vi "Command Formation And Communication.vi"(8 "error in (no error)":errorcluster, 9 "Command":string, 10 "Platform Slot Number":i16 min=-1 max=255, 11 "VISA resource name":refnum<visa-resource-name>) -> (0 "error out":errorcluster, 2 "Response":string, 3 "VISA resource name out":refnum<visa-resource-name>)   [LabVIEW 2018, in "LTB-1.lvlib" / "3150.lvlib"]
doc: "Responsible for communication with the device, sending the command and receiving the output, adding LINS keyword if command belongs to module-specific. Calls the error query based on the mode of communication and logged into the error cluster using Merge Error.vi if any error encounters."
uses:
  3150.lvlib
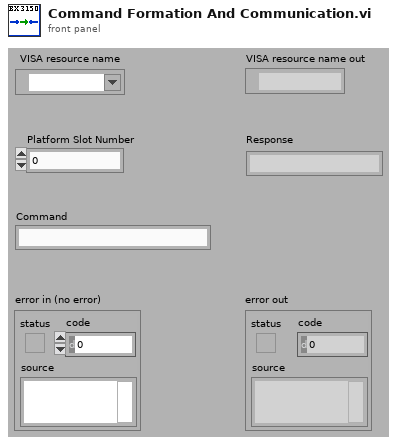
[diagram p1: front panel]
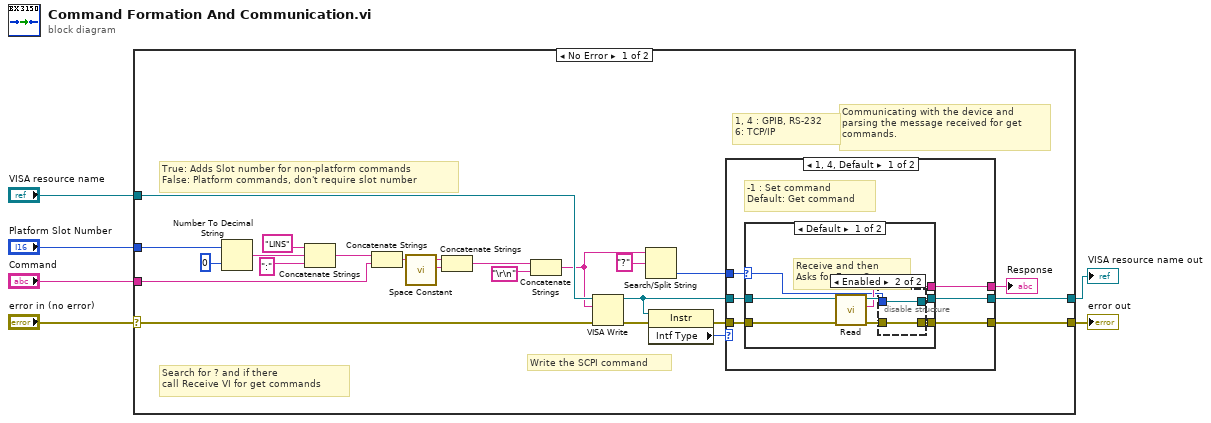
[diagram p0: block diagram]
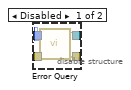
[diagram p2: hidden frame]
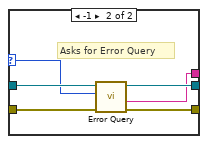
[diagram p3: hidden frame]
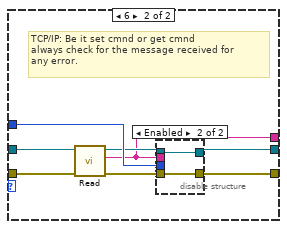
[diagram p4: hidden frame]
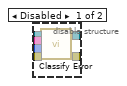
[diagram p5: hidden frame]
diagram:
  n1 = case shown="No Error" "error in (no error)" {
    selector: "error in (no error)" -> [w27 w73]
    tunnel: "VISA resource name" -> [w29 w74]
    tunnel: [w16 w74] -> w4
    tunnel: "Command" -> [w28 _]
    tunnel: [w15 w73] -> w1
    tunnel: "Platform Slot Number" -> [w26 _]
    frame No Error {
      # "1, 4 : GPIB, RS-232\n6: TCP/IP"
      # "Write the SCPI command"
      # "Search for ? and if there\ncall Receive VI for get commands"
      # "Communicating with the device and \nparsing the message received for get\ncommands."
      # "True: Adds Slot number for non-platform commands\nFalse: Platform commands, don't require slot number"
      n2 = Number To Decimal String(number=w26, width (-)=0) -> (decimal integer string=w9:string)
      n3 = Concatenate Strings("LINS", w9, ":" ("string")) -> (w10:string)
      n4 = Concatenate Strings(w10, w28) -> (w11:string)
      n5 = call <vilib>:"Space Constant.vi"() -> ("String"=w7:string)
      n6 = Concatenate Strings(w11, w7) -> (w25:string)
      n7 = Concatenate Strings(w25, "\r\n") -> (w22:string)
      n8 = VISA Write(VISA resource name=w29, write buffer=w22, error in (no error)=w27) -> (VISA resource name out=w19:refnum<visa-resource-name>, error out=w17:errorcluster)  [unwired: 1 out]
      n9 = Search/Split String(string=w22, search string/char (-)="?") -> (offset of match=w21:i32)  [unwired: 3 out]
      n10 = property class="Instr"(reference=w19, error in=w17) -> (error out=w18:errorcluster, "Intf Type"=w20:u16)  [unwired: 1 out]
      n11 = case shown="1, 4, Default" w20 {
        tunnel: w21 -> [w35 w62]
        tunnel: w19 -> [w33 w64]
        tunnel: w18 -> [w34 w63]
        tunnel: [w30 w59] -> w16
        tunnel: [w31 w58] -> w15
        tunnel: [w32 w57] -> w14
        frame 1, 4, Default {
          # "-1 : Set command\nDefault: Get command"
          n12 = case shown="Default" w35 {
            selector: w35 -> [w38 w51]
            tunnel: w34 -> [w43 w56]
            tunnel: w33 -> [w42 w55]
            tunnel: [w37 w54] -> w31
            tunnel: [w36 w53] -> w30
            tunnel: [w39 w52] -> w32
            frame Default {
              # "Receive and then \nAsks for Error Query"
              n13 = call "Read.vi"("error in (no error)"=w43, "VISA resource name"=w42) -> ("error out"=w40:errorcluster, "Message Received"=w39:string, "VISA resource name out"=w41:refnum<visa-resource-name>)  [unwired: 7 out]
              n14 = disable-structure shown="Enabled" {
                disable-tunnel: w41 -> [w48 w50]
                disable-tunnel: w40 -> [w47 w49]
                disable-tunnel: w38 -> [w46 _]
                disable-tunnel: [w45 w49] -> w37
                disable-tunnel: [w44 w50] -> w36
                frame Disabled {
                  n15 = call "Error Query.vi"("error in (no error)"=w47, "Command Type (0)"=w46, "VISA resource name"=w48) -> ("error out"=w45:errorcluster, "VISA resource name out"=w44:refnum<visa-resource-name>)  [unwired: 7 out]
                }
                frame Enabled {
                }
              }
            }
            frame -1 {
              # "Asks for Error Query"
              n16 = call "Error Query.vi"("error in (no error)"=w56, "Command Type (0)"=w51, "VISA resource name"=w55) -> ("error out"=w54:errorcluster, "Error Message"=w52:string, "VISA resource name out"=w53:refnum<visa-resource-name>)  [unwired: 6 out]
            }
          }
        }
        frame 6 {
          # "TCP/IP: Be it set cmnd or get cmnd\nalways check for the message received for\nany error."
          n17 = call "Read.vi"("error in (no error)"=w63, "VISA resource name"=w64) -> ("error out"=w60:errorcluster, "Message Received"=w57:string, "VISA resource name out"=w61:refnum<visa-resource-name>)  [unwired: 7 out]
          n18 = disable-structure shown="Enabled" {
            disable-tunnel: w62 -> [w70 _]
            disable-tunnel: w61 -> [w69 w72]
            disable-tunnel: w60 -> [w68 w71]
            disable-tunnel: [w67 w72] -> w59
            disable-tunnel: [w66 w71] -> w58
            disable-tunnel: w57 -> [w65 _]
            frame Disabled {
              n19 = call "Classify Error.vi"("error in (no error)"=w68, "Command Type (0)"=w70, "Message String"=w65, "VISA resource name"=w69) -> ("error out"=w66:errorcluster, "VISA resource name out"=w67:refnum<visa-resource-name>)  [unwired: 6 out]
            }
            frame Enabled {
            }
          }
        }
      }
      "Response" <- w14
    }
    frame Error {
    }
  }
  "VISA resource name out" <- w4
  "error out" <- w1
